vi "HB_SetLEDRGBValue.vi"(0 "HBDevRef":T1, 11 "error in (no error)":errorcluster, 12 "Red":u8, 13 "Green":u8, 14 "Blue":u8) -> (4 "HBDevRef":T1, 15 "error out":errorcluster)   [LabVIEW 2016]
doc: "Sets the color of the LEDs on the currently configured LED strip to the specified red, green, and blue values. Each value ranges from 0 to 255."
uses:
  <vilib>/Rock Robotics/WPI/SerialPort/WPI_SerialPortRef.ctl
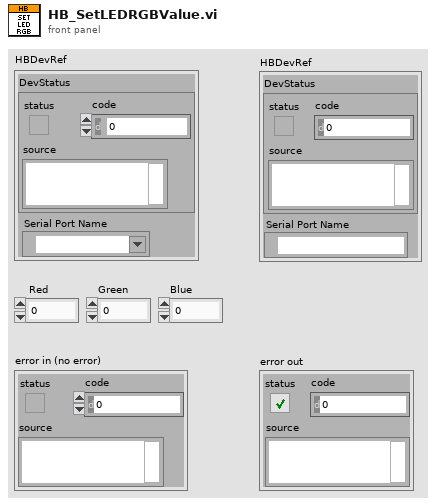
[diagram p1: front panel]
types:
  T1 = typedef "WPI_SerialPortRef.ctl" = cluster{"DevStatus":errorcluster, "Serial Port Name":refnum<visa-resource-name>}
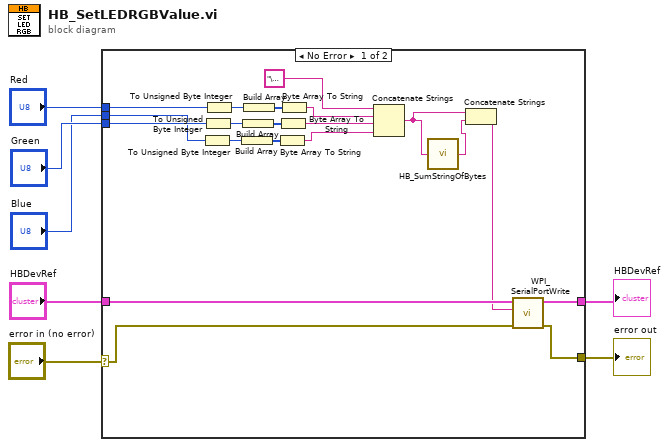
[diagram p0: block diagram]
diagram:
  n1 = case shown="No Error" "error in (no error)" {
    selector: "error in (no error)" -> [w8 w28]
    tunnel: "Red" -> [w27 _]
    tunnel: "Green" -> [w26 _]
    tunnel: "Blue" -> [w25 _]
    tunnel: "HBDevRef" -> [w24 w29]
    tunnel: [w23 w28] -> w3
    tunnel: [w22 w29] -> w2
    frame No Error {
      n2 = To Unsigned Byte Integer(number=w25) -> (unsigned 8bit integer=w17:u8)
      n3 = To Unsigned Byte Integer(number=w26) -> (unsigned 8bit integer=w19:u8)
      n4 = To Unsigned Byte Integer(number=w27) -> (unsigned 8bit integer=w21:u8)
      n5 = Build Array(w17) -> (w16:u8[])
      n6 = Build Array(w19) -> (w18:u8[])
      n7 = Build Array(w21) -> (w20:u8[])
      n8 = Byte Array To String(unsigned byte array=w16) -> (string=w15:string)
      n9 = Byte Array To String(unsigned byte array=w18) -> (string=w14:string)
      n10 = Byte Array To String(unsigned byte array=w20) -> (string=w13:string)
      n11 = Concatenate Strings("\u0015", w13, w14, w15) -> (w10:string)
      n12 = call "HB_SumStringOfBytes.vi"("String Of Bytes"=w10) -> ("Sum as String"=w9:string)
      n13 = Concatenate Strings(w10, w9) -> (w11:string)
      n14 = call <vilib>:"WPI_SerialPortWrite.vi"("error in (no error)"=w8, "Buffer"=w11, "SerialPortRef"=w24) -> ("error out"=w23:errorcluster, "SerialPortRef"=w22:T1)  [unwired: 6 in, 1 out]
    }
    frame Error {
    }
  }
  "error out" <- w3
  "HBDevRef" <- w2
